vi "oa_TV Extract Geometric Imperfection (Digital Tacho 1Chan).vi"(0 "digital tach info":T1={"tacho counts"=[], "counter timebase [Hz]"=20000000.0, "counter task type"=enum."event counting", "counter digit (32)"=32}, 3 "reset? (F)":bool, 7 "pulse/revolution":i32=1, 11 "error in (no error)":errorcluster) -> (4 "pulse positions":dbl[](array[numeric]), 8 "revulotion":i32, 10 "revulotion index":i32, 15 "error out":errorcluster)   [LabVIEW 2017, in "SoundVib_Torsional.lvlib"]
uses:
  <vilib>/addons/Sound and Vibration/Order Analysis/Torsional Vibration/SoundVib_Torsional.lvlib
  <vilib>/addons/Sound and Vibration/Order Analysis/Tach Process/SubVIs/digital tach info.ctl
  <vilib>/addons/Sound and Vibration/Order Analysis/Tach Process/SubVIs/oa_Process Counter Data (1 Tach).vi
  <vilib>/addons/Sound and Vibration/Order Analysis/Tach Process/SoundVib_TachProcess.lvlib
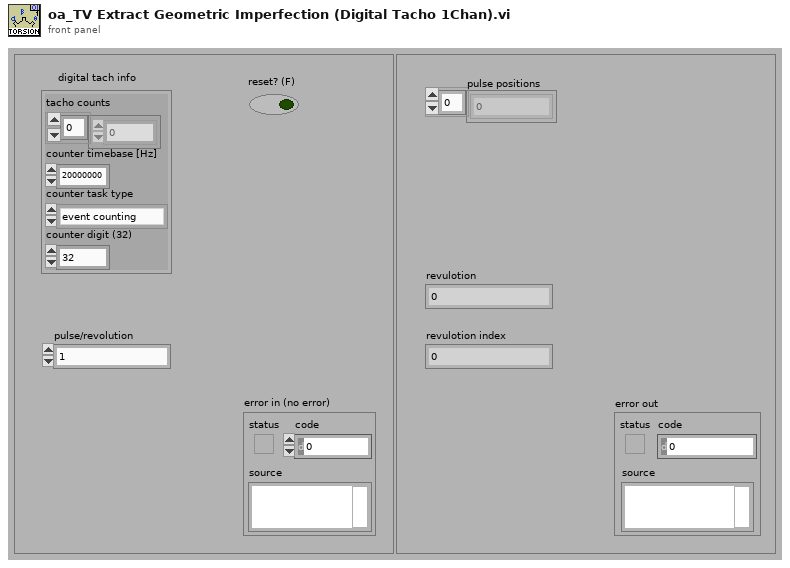
[diagram p1: front panel]
types:
  T1 = typedef "SoundVib_TachProcess.lvlib/digital tach info.ctl" = cluster{"tacho counts":i64[], "counter timebase [Hz]":dbl, "counter task type":enum16{"period measurement", "event counting"}, "counter digit (32)":i32}
  T2 = cluster{"pulse positions [s]":dbl[], "counter timebase [Hz]":dbl, "counter task type":enum16{"period measurement", "event counting"}, "counter digit":i32}
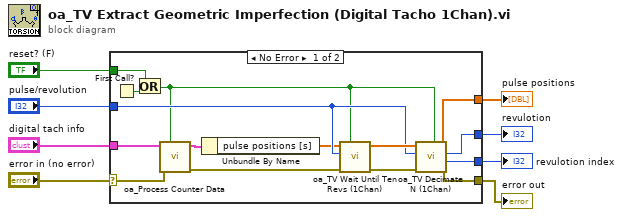
[diagram p0: block diagram]
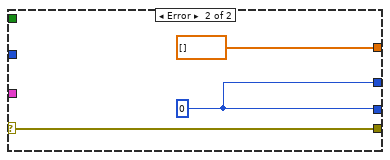
[diagram p2: hidden frame]
diagram:
  n1 = case shown="No Error" "error in (no error)" {
    selector: "error in (no error)" -> [w19 w26]
    tunnel: "pulse/revolution" -> [w14 _]
    tunnel: [w21 dbl[] [] ("Array")] -> w7
    tunnel: [w23 w25] -> w6
    tunnel: [w22 w25] -> w5
    tunnel: [w10 w26] -> w3
    tunnel: "digital tach info" -> [w20 _]
    tunnel: "reset? (F)" -> [w11 _]
    frame No Error {
      n2 = First Call?() -> (First Call?: T/F=w12:bool)
      n3 = Or(x=w11, y=w12) -> (x .or. y?=w13:bool)
      n4 = call-poly <vilib>:"oa_Process Counter Data.vi"("reset?(True)"=w13, "error in (no error)"=w19, "digital tach info"=w20) -> ("error out (no error)"=w17:errorcluster, "digital tach info (DBL)"=w18:T2)  [unwired: 7 in]
      n5 = Unbundle By Name(w18) -> ("pulse positions [s]"=w9:dbl[])
      n6 = call <vilib>:"oa_TV Wait Until Ten Revs (1Chan).vi"("reset? (F)"=w13, "error in (no error)"=w17, "pulse/revolution"=w14, "pulse positions"=w9) -> ("error out"=w16:errorcluster, "pulse positions out"=w15:dbl[])  [unwired: 6 in]
      n7 = call <vilib>:"oa_TV Decimate N (1Chan).vi"("reset? (F)"=w13, "error in (no error)"=w16, "pulse/revolution"=w14, "pulse positions [s]"=w15) -> ("error out"=w10:errorcluster, "revolution index"=w22:i32, "revolution"=w23:i32, "pulse positions"=w21:dbl[])  [unwired: 4 in]
    }
    frame Error {
      w25 = 0 ("Revulotion")
    }
  }
  "revulotion" <- w6
  "pulse positions" <- w7
  "revulotion index" <- w5
  "error out" <- w3
